vi "Model - DeInit.vi"(8 "error in (no error)":errorcluster, 11 "View Model":T1) -> (0 "error out":errorcluster)   [LabVIEW 2017]
doc: "De-Initialize all components of View Model."
uses:
  Controls/View Model.ctl
  Controls/Shared Model.ctl
  Error Handler/Controls/Error Model.ctl
  Error Handler/Controls/Error Data.ctl
  Error Handler/Controls/Error Level.ctl
  Configuration/Controls/Config Model.ctl
  Configuration/Controls/Config Data Record.ctl
  Configuration/Controls/Config Command.ctl
  Controller/Controls/Control Model.ctl
  Controller/Controls/Elevator Location.ctl
  Controller/Controls/Elevator Status.ctl
  Controller/Controls/Control Event.ctl
  Controller/Controls/Control CMD.ctl
  Controller/Controls/Controller - Overhead.ctl
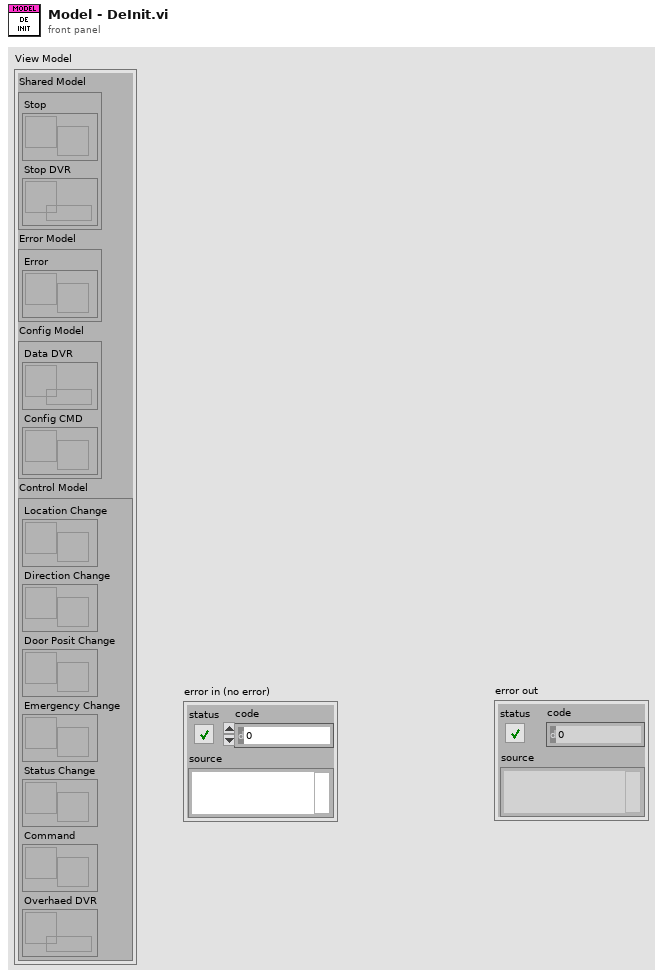
[diagram p1: front panel]
types:
  T1 = typedef "View Model.ctl" = cluster{"Shared Model":T2, "Error Model":T3, "Config Model":T4, "Control Model":T5}
  T2 = typedef "Shared Model.ctl" = cluster{"Stop":refnum<user-event>, "Stop DVR":refnum<data-value>}
  T3 = typedef "Error Model.ctl" = cluster{"Error":refnum<user-event>}
  T4 = typedef "Config Model.ctl" = cluster{"Data DVR":refnum<data-value>, "Config CMD":refnum<user-event>}
  T5 = typedef "Control Model.ctl" = cluster{"Location Change":refnum<user-event>, "Direction Change":refnum<user-event>, "Door Posit Change":refnum<user-event>, "Emergency Change":refnum<user-event>, "Status Change":refnum<user-event>, "Command":refnum<user-event>, "Overhaed DVR":refnum<data-value>}
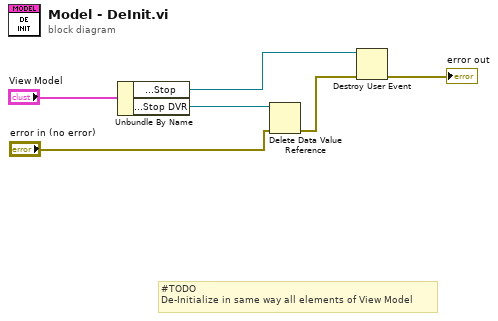
[diagram p0: block diagram]
diagram:
  # "#TODO\nDe-Initialize in same way all elements of View Model"
  n1 = Unbundle By Name("View Model") -> ("Shared Model.Stop"=w5:refnum<user-event>, "Shared Model.Stop DVR"=w4:refnum<data-value>)
  n2 = Delete Data Value Reference(data value reference=w4, error in="error in (no error)") -> (error out=w2:errorcluster)  [unwired: 1 out]
  n3 = Destroy User Event(user event=w5, error in=w2) -> (error out=→"error out":errorcluster)
